vi "PowerSupplyControlVoltageMode.vi"(4 "OnOff":bool, 5 "Max Current (A)":dbl=1.0, 6 "Z-":dbl, 7 "X+":dbl, 8 "Z+":dbl, 9 "Y-":dbl, 10 "Y+":dbl, 11 "X-":dbl) -> (0 "Saturating":bool, 3 "Max Current":dbl)   [LabVIEW 2017]
uses:
  <vilib>/imath/engines/lvmath2/RunTimeEngine/Managers/WorkSpace/UID Generator.vi
  <vilib>/imath/engines/lvmath2/RunTimeEngine/BuiltInFunctions/abs/NIMS_abs(signed).vi
  <instcachedir>/0/NIMS_abs(signed)_C4FCB8E6058B49B797C7C8D53CA5F6EC.lvgen/NIMS_abs(signed)_C4FCB8E6058B49B797C7C8D53CA5F6EC_001.vi
  <vilib>/imath/engines/lvmath2/RunTimeEngine/BuiltInFunctions/max/1 input/NIMS_max(RV).vi
  <instcachedir>/0/NIMS_max(RV)_237633DB1D604D5BA7001287DF3C7957.lvgen/NIMS_max(RV)_237633DB1D604D5BA7001287DF3C7957_000.vi
  <vilib>/imath/engines/lvmath2/RunTimeEngine/RunTimeType/NIMS_RunTimeType_From StrictType (excl LVString).vi
  <instcachedir>/0/NIMS_RunTimeType_From StrictType (excl LVString)_1019F277F0A747EDBCA0F6C52CA54500.lvgen/NIMS_RunTimeType_From StrictType (excl LVString)_1019F277F0A747EDBCA0F6C52CA54500_000.vi
  <vilib>/imath/engines/lvmath2/RunTimeEngine/LocalVariableDefStatement/MC_LocalVariableDefStatement_Display.vi
  <vilib>/imath/engines/lvmath2/RunTimeEngine/RunTimeType/NIMS_RunTimeType_Set Source Original Bool.vi
  <vilib>/imath/engines/lvmath2/RunTimeEngine/IndexRead/NIMS V(S).vi
  <instcachedir>/0/NIMS V(S)_0488751826AF41519A22953C041130DC.lvgen/NIMS V(S)_0488751826AF41519A22953C041130DC_000.vi
  <vilib>/imathl/engines/lvmath/Functions/Error Handling/Create Error.vi
  <vilib>/imath/engines/lvmath2/RunTimeEngine/Managers/SymbolTable/Clear UID.vi
  <vilib>/imath/engines/lvmath2/RunTimeEngine/NodeEndStatement/NIMS_NodeEndStatement_Output.vi
  <instcachedir>/0/NIMS_NodeEndStatement_Output_53EC0D466D134D7ABD903AC30B43404B.lvgen/NIMS_NodeEndStatement_Output_53EC0D466D134D7ABD903AC30B43404B_001.vi
  <instcachedir>/0/NIMS_NodeEndStatement_Output_53EC0D466D134D7ABD903AC30B43404B.lvgen/NIMS_NodeEndStatement_Output_53EC0D466D134D7ABD903AC30B43404B_010.vi
  <vilib>/imath/engines/lvmath2/RunTimeEngine/ErrorHandling/NIMS_Finalize Error.vi
  <vilib>/imath/engines/lvmath2/RunTimeEngine/Managers/SymbolTable/NIMS_WorkSpace.lvlib
panel:
  out "Waveform Chart":dbl(graph)
  # "Currents setpoint"
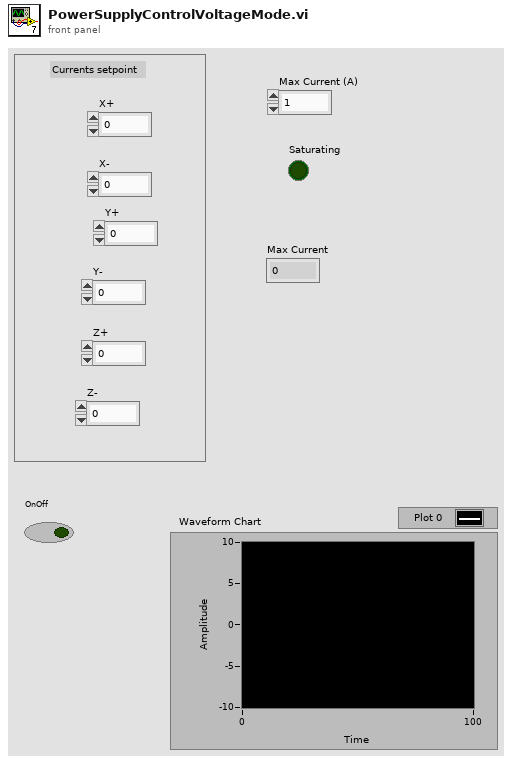
[diagram p1: front panel]
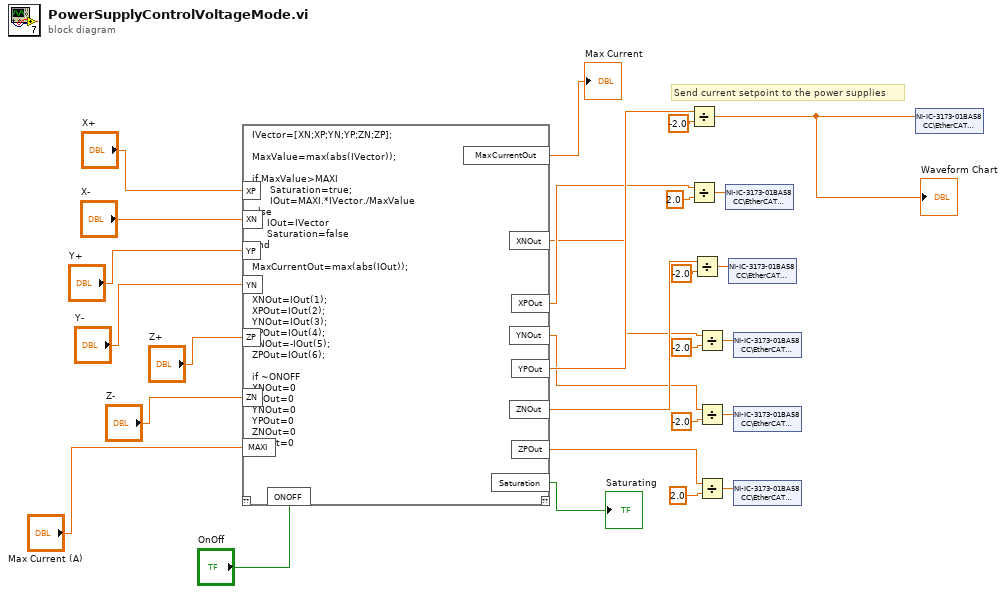
[diagram p0: block diagram]
diagram:
  # "Send current setpoint to the power supplies"
  n1 = mathscript code="IVector=[XN;XP;YN;YP;ZN;ZP];\n\nMaxValue=max(abs(IVector));\n\nif MaxValue>MAXI\n      Saturation=true;\n      IOut=MAXI.*IVector./MaxValue\nelse\n     IOut=IVector\n     Saturation=false\nend\n\nMaxCurrentOut=max(abs(IOut));\n\n\nXNOut=IOut(1);\nXPOut=IOut(2);\nYNOut=IOut(3);\nYPOut=IOut(4);\nZNOut=-IOut(5);\nZPOut=IOut(6);\n\nif ~ONOFF\nXNOut=0\nXPOut=0\nYNOut=0\nYPOut=0\nZNOut=0\nZPOut=0\nend"("YP"="Y+", "YN"="Y-", "XP"="X+", "XN"="X-", "ZP"="Z+", "ZN"="Z-", "MAXI"="Max Current (A)", "ONOFF"="OnOff") -> ("XNOut"=w7:dbl, "XPOut"=w9:dbl, "YNOut"=w6:dbl, "YPOut"=w10:dbl, "ZNOut"=w8:dbl, "ZPOut"=w5:dbl, "Saturation"=→"Saturating":bool, "MaxCurrentOut"=→"Max Current":dbl)  [unwired: 1 in, 1 out]
  n2 = Divide(x=w10, y=-2.0) -> (x/y=w2:dbl)
  "Waveform Chart" <- w2
  n3 = Divide(x=w9, y=2.0) -> (x/y=w22:dbl)
  n4 = Divide(x=w8, y=-2.0) -> (x/y=w27:dbl)
  n5 = Divide(x=w7, y=-2.0) -> (x/y=w25:dbl)
  n6 = Divide(x=w6, y=-2.0) -> (x/y=w21:dbl)
  n7 = Divide(x=w5, y=2.0) -> (x/y=w19:dbl)
  n8 = shared-variable "NI-IC-3173-01BA58CC\\EtherCAT Master\\Device\\Mod1\\AO0"(w22) -> ()  [unwired: 1 in, 1 out]
  n9 = shared-variable "NI-IC-3173-01BA58CC\\EtherCAT Master\\Device\\Mod1\\AO1"(w27) -> ()  [unwired: 1 in, 1 out]
  n10 = shared-variable "NI-IC-3173-01BA58CC\\EtherCAT Master\\Device\\Mod1\\AO3"(w25) -> ()  [unwired: 1 in, 1 out]
  n11 = shared-variable "NI-IC-3173-01BA58CC\\EtherCAT Master\\Device\\Mod1\\AO2"(w21) -> ()  [unwired: 1 in, 1 out]
  n12 = shared-variable "NI-IC-3173-01BA58CC\\EtherCAT Master\\Device\\Mod2\\AO1"(w19) -> ()  [unwired: 1 in, 1 out]
  n13 = shared-variable "NI-IC-3173-01BA58CC\\EtherCAT Master\\Device\\Mod2\\AO0"(w2) -> ()  [unwired: 1 in, 1 out]
